vi "sub_center_pt.vi"(10 "point-2":cluster{"x":dbl, "y":dbl}, 11 "point-1":cluster{"x":dbl, "y":dbl}) -> (3 "center":cluster{"x":dbl, "y":dbl})   [LabVIEW 2019]
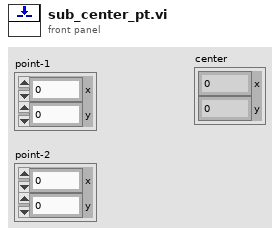
[diagram p1: front panel]
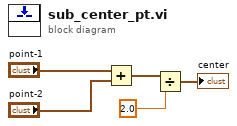
[diagram p0: block diagram]
diagram:
  n1 = Add(x="point-1", y="point-2") -> (x+y=w4:cluster{"x":dbl, "y":dbl})
  n2 = Divide(x=w4, y=2.0) -> (x/y=→"center":cluster{"x":dbl, "y":dbl})
